vi "New.vi"(8 "Error In":errorcluster, 11 "String":string) -> (0 "Error Out":errorcluster, 3 "String":refnum<class "String.lvclass">)   [LabVIEW 2018, in "Toolkit.lvlib" / "Readers.lvlib" / "String.lvclass"]
uses:
  String.lvclass
  String.lvclass/String.ctl
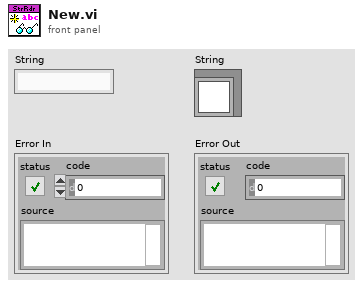
[diagram p1: front panel]
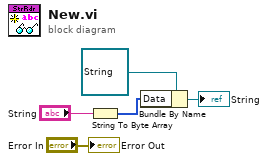
[diagram p0: block diagram]
diagram:
  n1 = String To Byte Array(string="String") -> (unsigned byte array=w3:u8[])
  n2 = Bundle By Name(cluster=refnum<class "String.lvclass"> refnum ("Mustache.lvlib:Readers.lvlib:String.lvclass"), "Data"=w3) -> (→"String":refnum<class "String.lvclass">)
  "Error Out" <- "Error In"
